vi "CANopenReadEncoder.vi"() -> ()   [LabVIEW 2020]
uses:
  <vilib>/Platform/TimedLoop/XDataNode/timing_clust.ctl
  <vilib>/Platform/TimedLoop/XDataNode/nitl_modes.ctl
  <vilib>/Platform/TimedLoop/XDataNode/wakeup.ctl
  <vilib>/CANopenLib/CANOPEN.llb/CANopen Interface Create.vi
  <vilib>/CANopenLib/CANOPEN.llb/CANopen TPDO Create.vi
  <vilib>/CANopenLib/CANOPEN.llb/CANopen TPDO Start.vi
  <vilib>/CANopenLib/CANOPEN.llb/CANopen SDO Create.vi
  <vilib>/CANopenLib/CANOPEN.llb/CANopen SDO Write [I16].vi
  <vilib>/CANopenLib/CANOPEN.llb/CANopen SDO Close.vi
  <vilib>/CANopenLib/CANOPEN.llb/CANopen SYNC Create.vi
  <vilib>/CANopenLib/CANOPEN.llb/CANopen RPDO Create.vi
  <vilib>/CANopenLib/CANOPEN.llb/CANopen SYNC Start.vi
  <vilib>/CANopenLib/CANOPEN.llb/CANopen RPDO Start.vi
  <vilib>/CANopenLib/CANOPEN.llb/CANopen Fetch from Data [U32].vi
  <vilib>/CANopenLib/CANOPEN.llb/CANopen TPDO Close.vi
  <vilib>/CANopenLib/CANOPEN.llb/CANopen Interface Close.vi
  <vilib>/CANopenLib/CANOPEN.llb/CANopen Convert To Data [I16].vi
  <vilib>/CANopenLib/CANOPEN.llb/CANopen Fetch from Data [I16].vi
  <vilib>/CANopenLib/CANOPEN.llb/CANopen Fetch from Data [I32].vi
  <vilib>/CANopenLib/CANOPEN.llb/CANopen SYNC Close.vi
  <vilib>/CANopenLib/CANOPEN.llb/CANopen RPDO Close.vi
  <vilib>/Platform/TimedLoop/XDataNode/XDataNode.xnode
  <vilib>/Platform/TimedLoop/XDataNode/XDNodeRunTimeDep.lvlib
panel:
  out "Target_Speed2":dbl
  out "Target_Speed1":dbl
  out "completion code 5":u32
  in  "buffer size (0) 7":u16
  in  "TPDO channel 2":u8(ring)=2 items=["PDO 1", "PDO 2", "PDO 3", "PDO 4"]
  in  "Set Target Vilocity 2":i16
  in  "stop 5":bool
  out "timestamp 5":timestamp=timestamp(3829477264.1142135 s since 1904-01-01)
  out "电机绝对位置 2":i32=2114697600
  out "速度反馈值 2":i32
  out "转矩反馈值 0.1% 2":i16=-28
  in  "buffer size (0) 6":u16=10
  in  "TPDO channel read 2":u8(ring)=1 items=["PDO 1", "PDO 2", "PDO 3", "PDO 4"]
  in  "RPDO channel write 2":u8(ring)=1 items=["PDO 1", "PDO 2", "PDO 3", "PDO 4"]
  in  "period (ms) 5":i64=10
  out "completion code 4":u32
  out "completion code 3":u32
  in  "batch SDO name 2":string="Nimotion_VM"
  in  "node-ID  2":u8=2 min=1 max=127 step=1
  out "completion code":u32
  in  "buffer size (0) 5":u16
  in  "TPDO channel":u8(ring)=2 items=["PDO 1", "PDO 2", "PDO 3", "PDO 4"]
  in  "Set Target Vilocity":i16
  in  "stop 4":bool
  out "timestamp 4":timestamp=timestamp(3829477264.1140933 s since 1904-01-01)
  out "电机绝对位置":i32=-1267158272
  out "速度反馈值":i32
  out "转矩反馈值 0.1%":i16=-12
  in  "buffer size (0) 4":u16=10
  in  "TPDO channel read":u8(ring)=1 items=["PDO 1", "PDO 2", "PDO 3", "PDO 4"]
  in  "RPDO channel write":u8(ring)=1 items=["PDO 1", "PDO 2", "PDO 3", "PDO 4"]
  in  "period (ms) 4":i64=10
  out "completion code 2":u32
  out "completion code 1":u32
  in  "batch SDO name":string="Nimotion_VM"
  in  "node-ID  4":u8=1 min=1 max=127 step=1
  in  "baud rate 2":u32(ring) items=["1 Mbit/s"=0, "800 kbit/s"=1, "500 kbit/s"=2, "250 kbit/s"=3, "125 kbit/s"=4, "50 kbit/s"=6, "20 kbit/s"=7, "10 kbit/s"=8]
  in  "CANopen interface 2":u32(ring) items=["CANopen01", "CANopen02", "CANopen03", "CANopen04", "CANopen05", "CANopen06", "CANopen07", "CANopen08", "CANopen09", "CANopen10", "CANopen11", "CANopen12", "CANopen13", "CANopen14", "CANopen15", "CANopen16", "CANopen17", "CANopen18", "CANopen19", "CANopen20", "CANopen21", "CANopen22", "CANopen23", "CANopen24", "CANopen25", "CANopen26", "CANopen27", "CANopen28", "CANopen29", "CANopen30", "CANopen31", "CANopen32"]
  in  "buffer size (0) 3":u16=10
  in  "period (ms) 3":i64=1
  in  "stop 3":bool
  out "New data? 3":bool
  out "timestamp 3":timestamp
  out "当前位置 3":u32
  out "基座原始角度值":dbl
  out "TPDO Data 3":u8[](array[numeric])
  out "基座角度值":dbl
  in  "PDO channel 3":u8(ring) items=["PDO 1", "PDO 2", "PDO 3", "PDO 4"]
  in  "node-ID 3":u8=3 min=1 max=127 step=1
  in  "buffer size (0) 2":u16=10
  in  "period (ms) 2":i64=1
  in  "stop 2":bool
  out "New data? 2":bool
  out "timestamp 2":timestamp
  out "当前位置 2":u32
  out "大臂原始角度值":dbl
  out "TPDO Data 2":u8[](array[numeric])
  out "大臂角度值":dbl
  in  "PDO channel 2":u8(ring) items=["PDO 1", "PDO 2", "PDO 3", "PDO 4"]
  in  "node-ID 2":u8=2 min=1 max=127 step=1
  out "三角形角度":dbl
  out "手腕角度值":dbl
  out "TPDO Data":u8[](array[numeric])
  out "手腕原始角度值":dbl
  out "当前位置":u32
  in  "buffer size (0)":u16=10
  in  "period (ms)":i64=1
  in  "stop":bool
  out "New data?":bool
  out "timestamp":timestamp
  in  "PDO channel":u8(ring) items=["PDO 1", "PDO 2", "PDO 3", "PDO 4"]
  in  "node-ID":u8=1 min=1 max=127 step=1
  in  "baud rate":u32(ring)=2 items=["1 Mbit/s"=0, "800 kbit/s"=1, "500 kbit/s"=2, "250 kbit/s"=3, "125 kbit/s"=4, "50 kbit/s"=6, "20 kbit/s"=7, "10 kbit/s"=8]
  in  "CANopen interface":u32(ring)=2 items=["CANopen01", "CANopen02", "CANopen03", "CANopen04", "CANopen05", "CANopen06", "CANopen07", "CANopen08", "CANopen09", "CANopen10", "CANopen11", "CANopen12", "CANopen13", "CANopen14", "CANopen15", "CANopen16", "CANopen17", "CANopen18", "CANopen19", "CANopen20", "CANopen21", "CANopen22", "CANopen23", "CANopen24", "CANopen25", "CANopen26", "CANopen27", "CANopen28", "CANopen29", "CANopen30", "CANopen31", "CANopen32"]
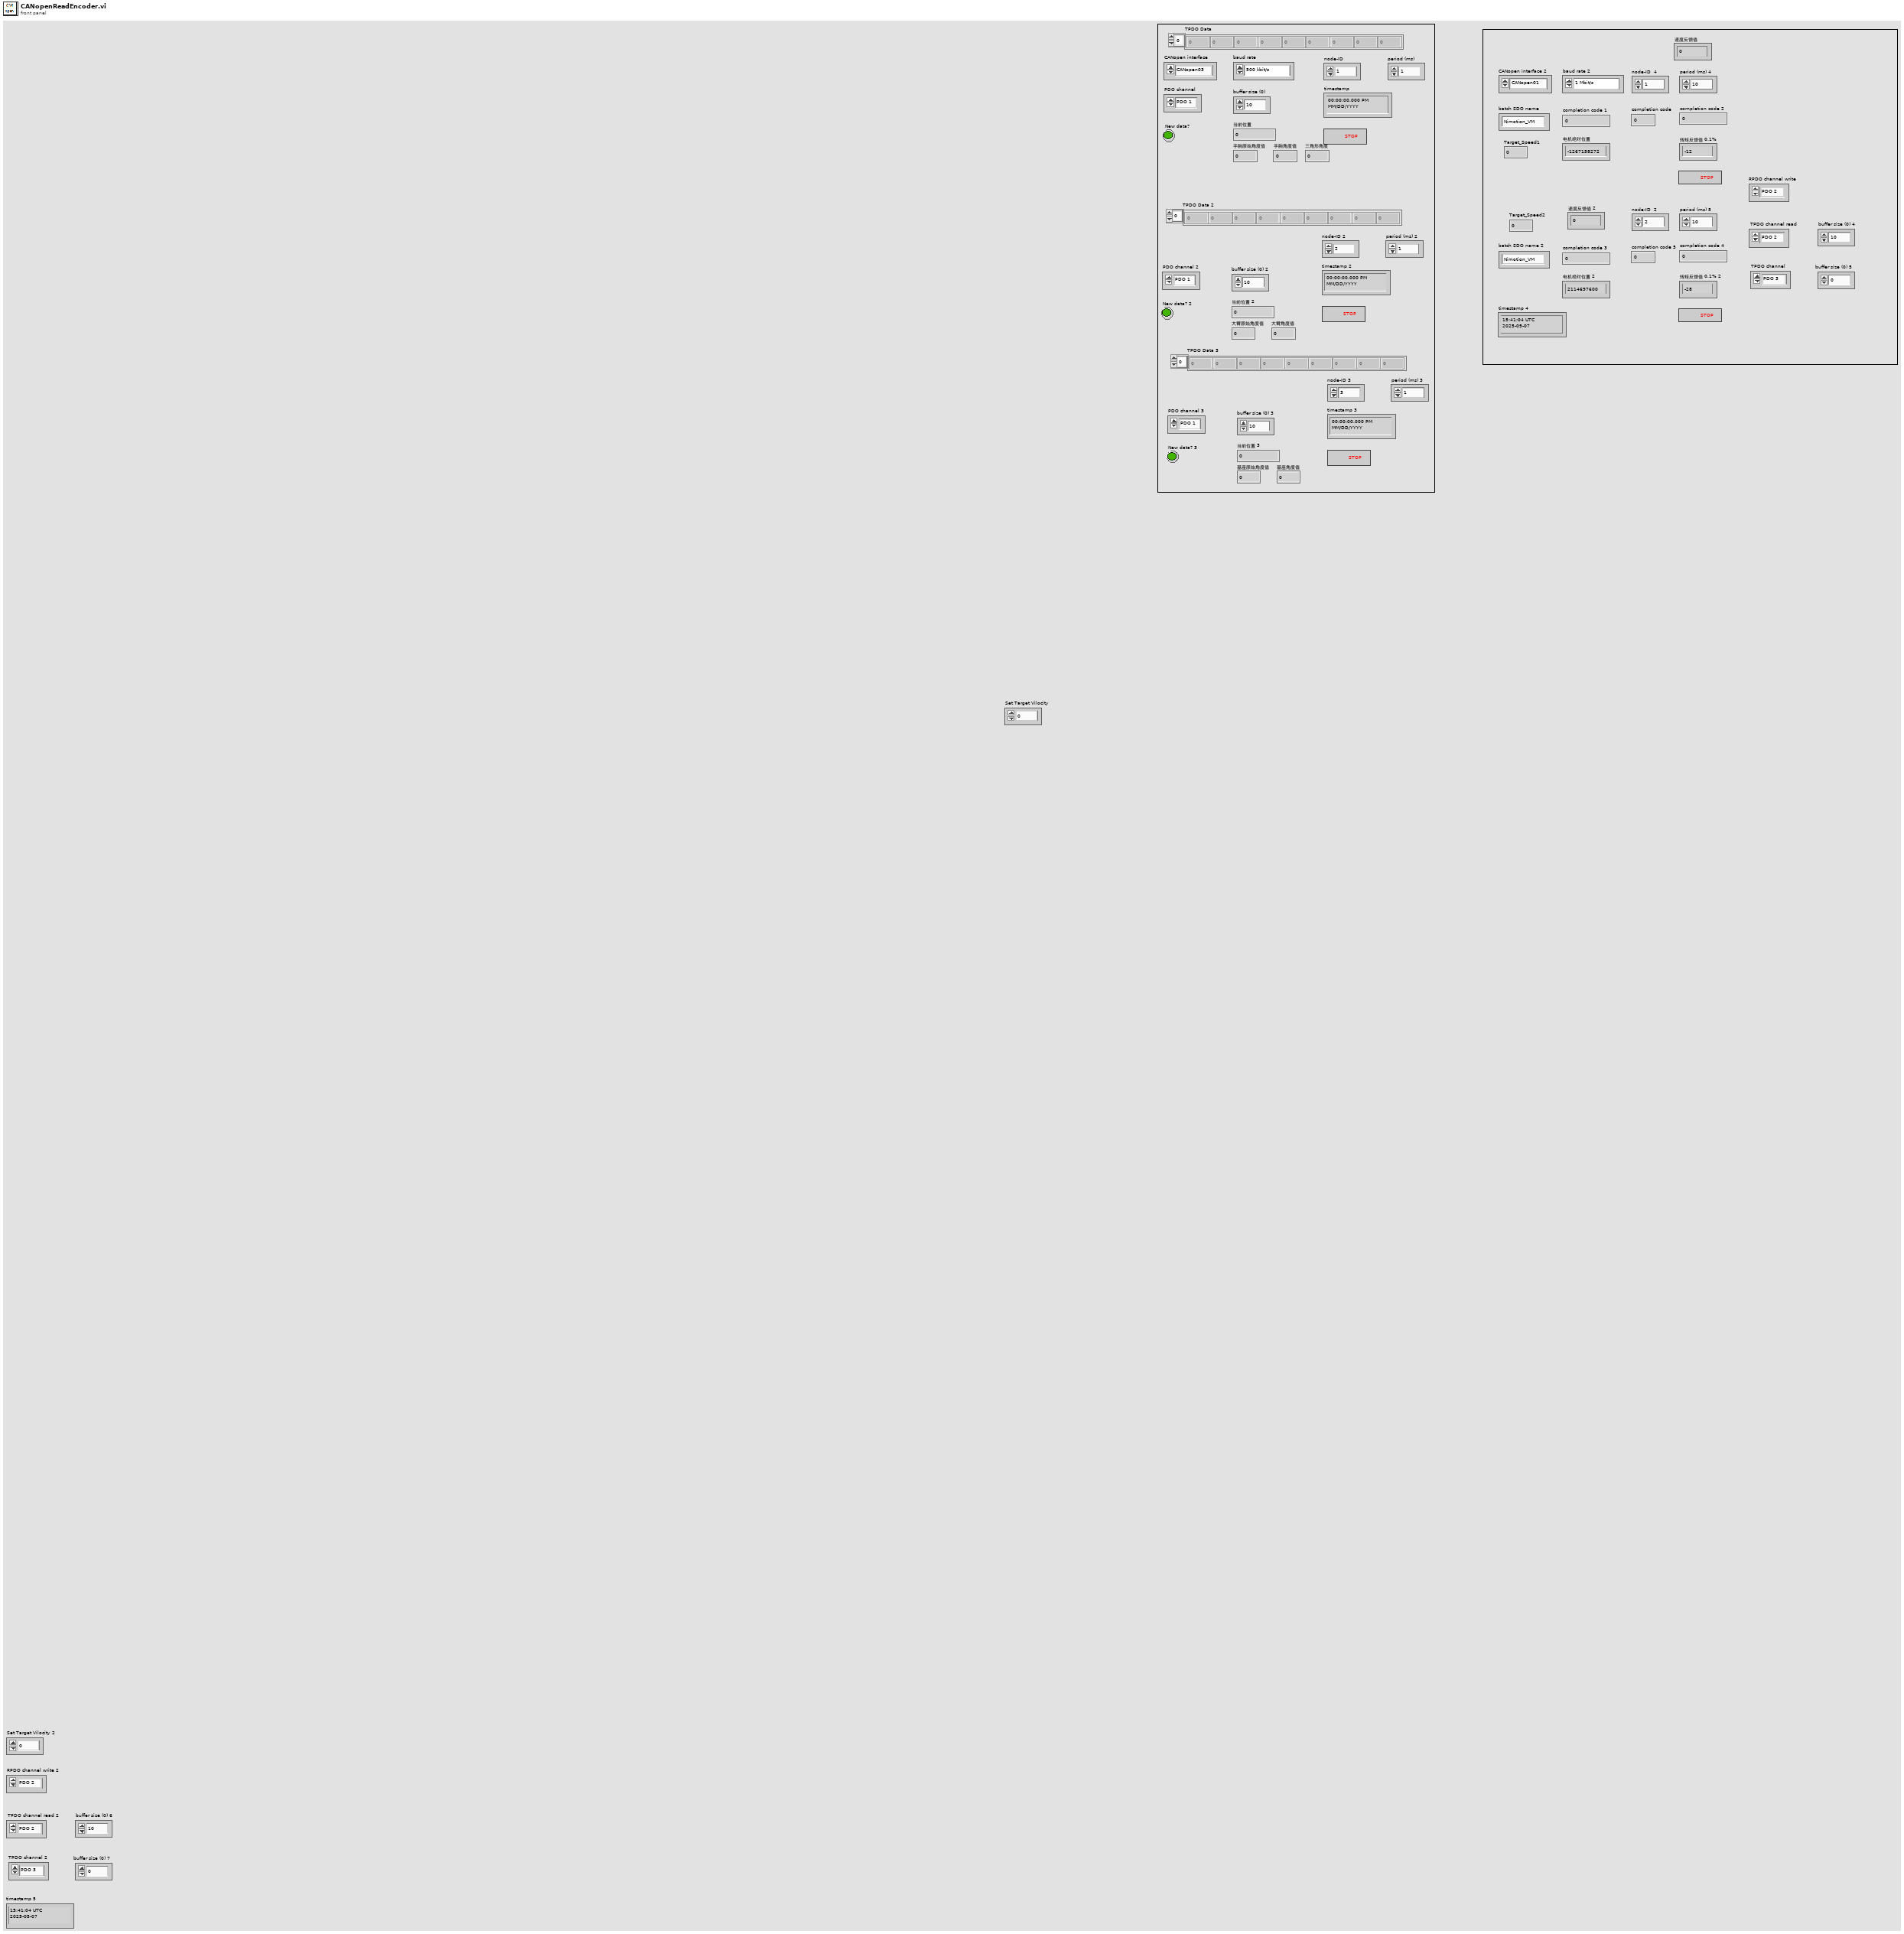
[diagram p1: front panel]
types:
  T1 = typedef "XDNodeRunTimeDep.lvlib/timing_clust.ctl" = cluster{"Expected End [f-1]":u64, "Actual End [f-1]":u64, "Finished Late? [f-1]":bool, "Expected End [i-1]":u64, "Actual End [i-1]":u64, "Finished Late? [i-1]":bool, "Expected Start [i]":u64, "Actual Start [i]":u64, "Expected Start [f]":u64, "Actual Start [f]":u64, "Source Name":string, "Structure Name":string, "Period":i64, "Deadline":i64, "Offset":i64, "Start":i64, "Priority":i32, "Timeout":i32, "Mode":T2, "Wakeup Reason":T3, "Error":errorcluster, "Source Type":string, "Secondary Source Type":string, "Global End Time":u64, "Global Start Time":u64, "Frame Duration":u64, "Iteration Duration":u64, "Assigned CPU":i32, "I/O Scan Engine Mode":u32}
  T2 = typedef "XDNodeRunTimeDep.lvlib/nitl_modes.ctl" = enum32{"No Change", "Process missed periods, maintain original phase", "Discard missed periods, maintain original phase", "Process missed periods, ignore original phase", "Discard missed periods, ignore original phase"}
  T3 = typedef "XDNodeRunTimeDep.lvlib/wakeup.ctl" = enum32{"Normal", "Aborted", "Asynchronous wakeup", "Timing source error", "Timed loop error", "Timeout"}
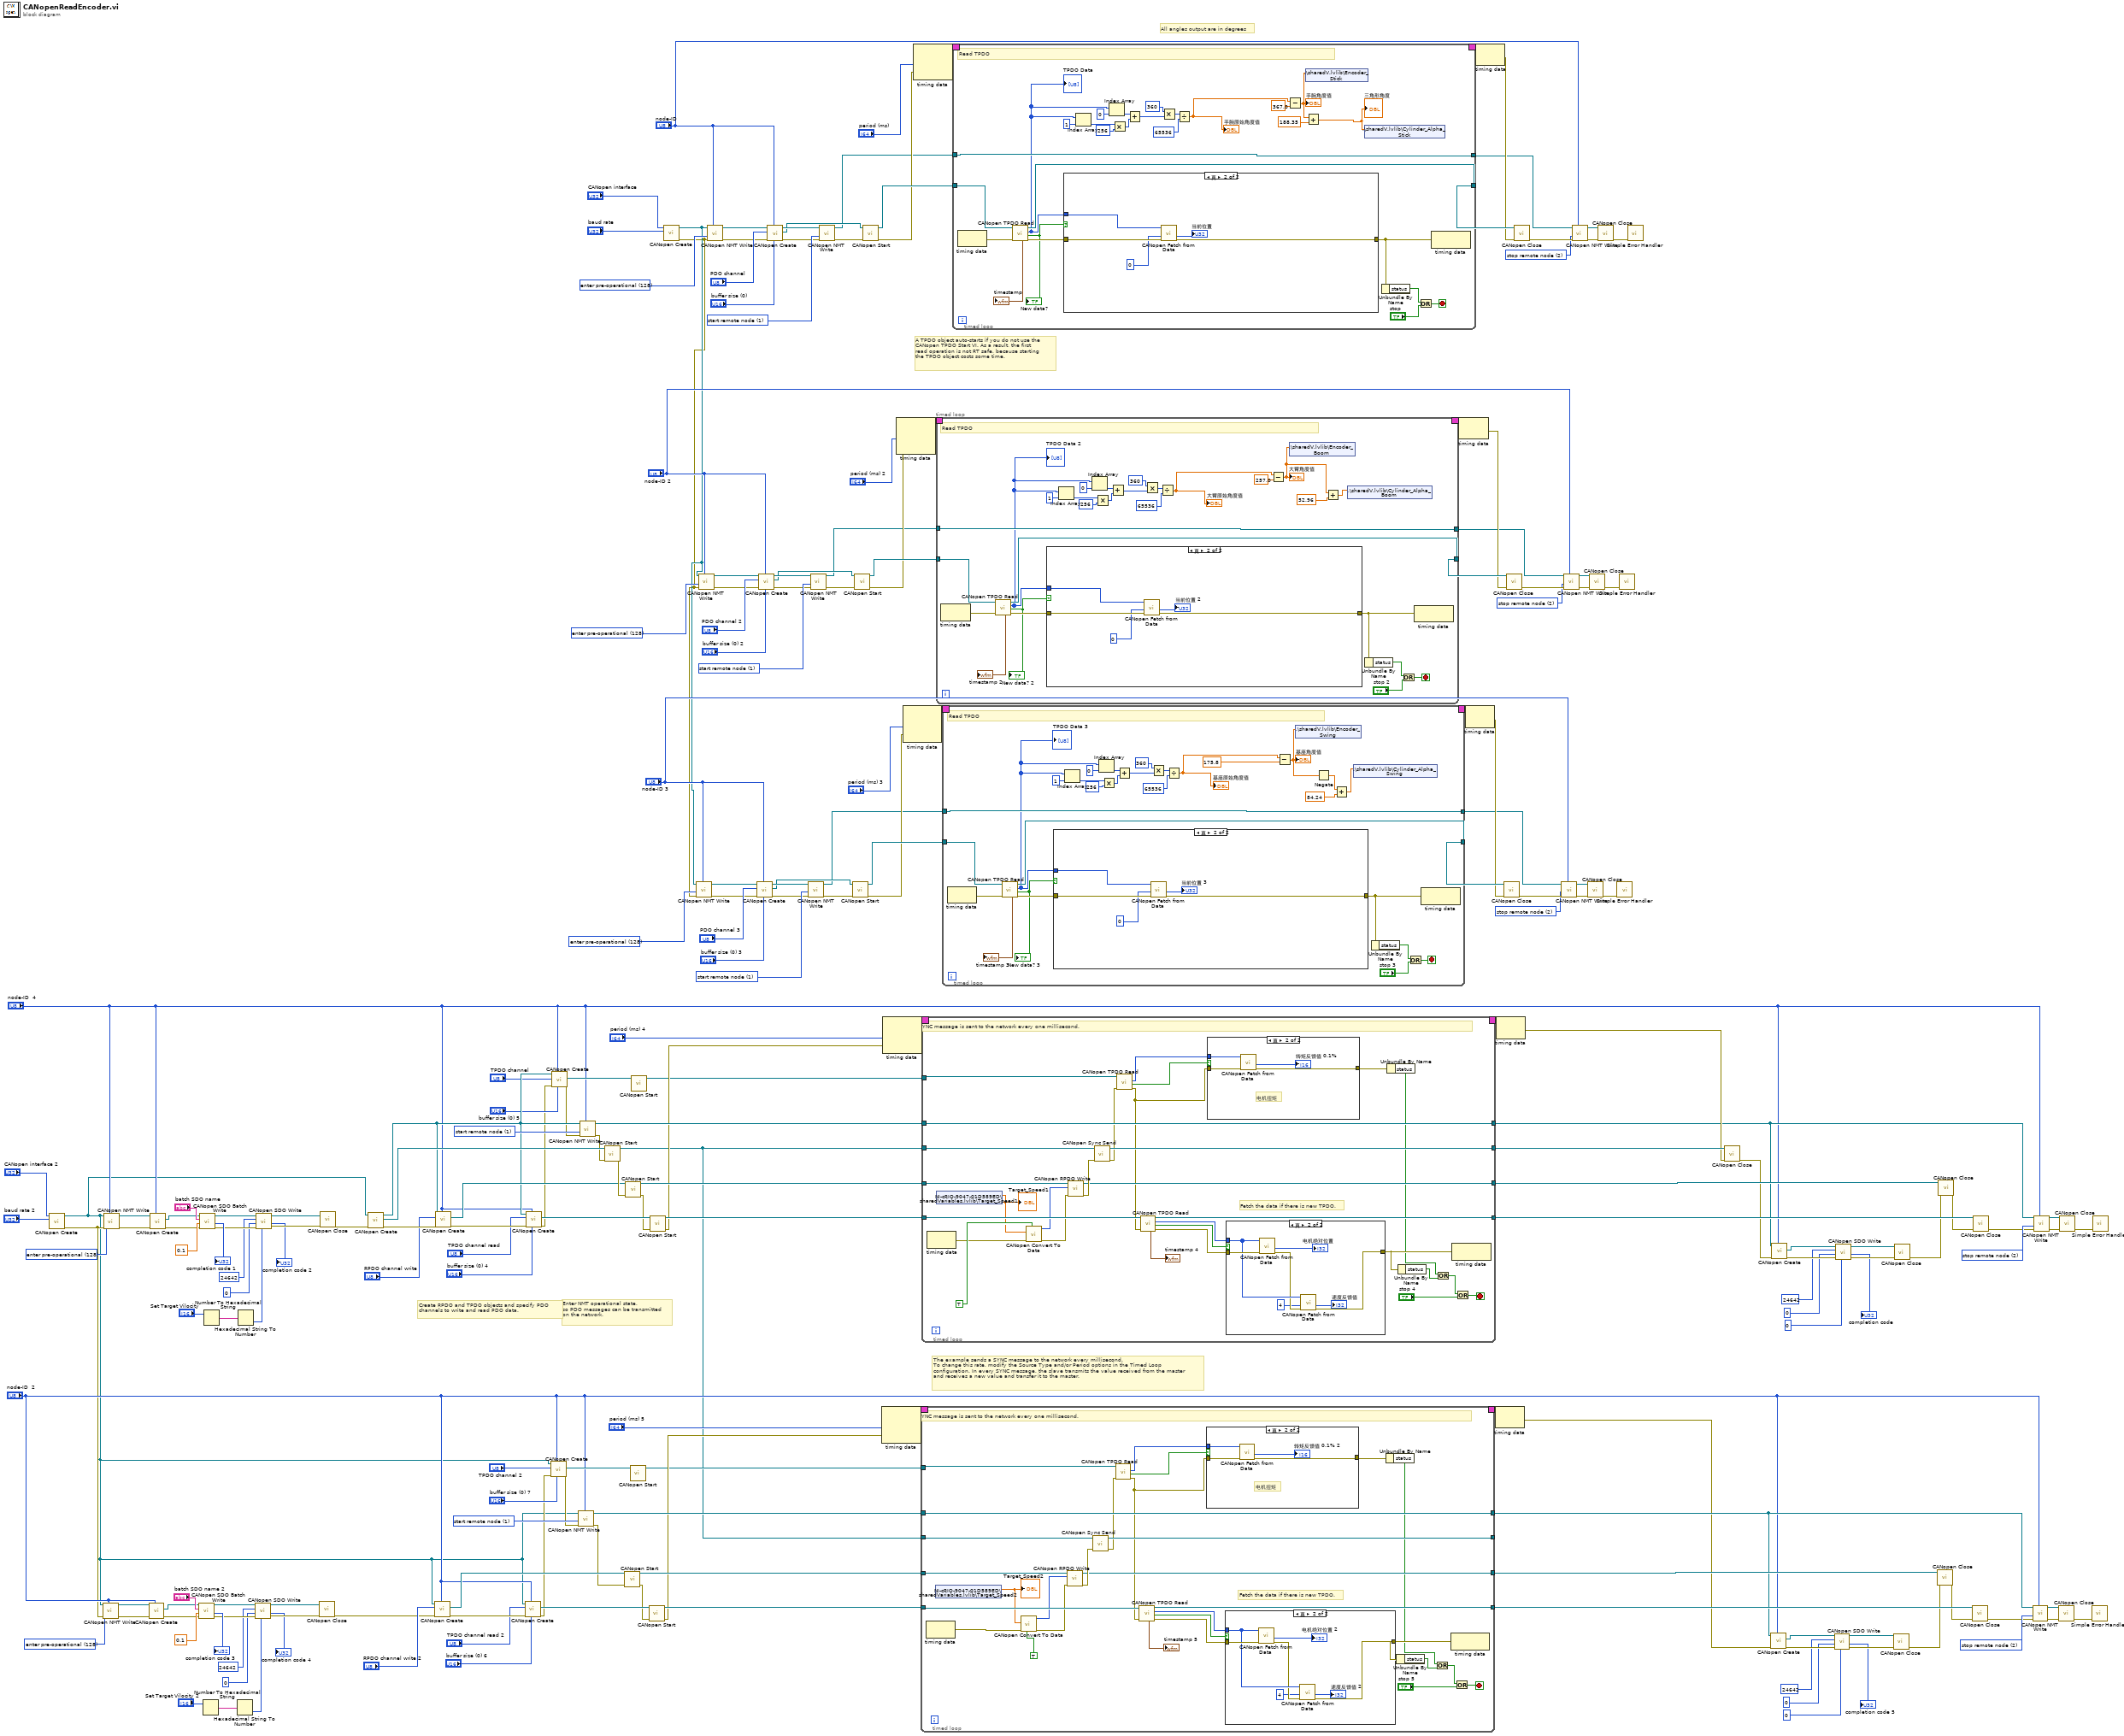
[diagram p0: block diagram]
diagram:
  w38 = u16 2 items=["start remote node"=1, "stop remote node"=2, "enter pre-operational"=128, "reset node"=129, "reset communication"=130] ("command")
  w46 = u16 1 items=["start remote node"=1, "stop remote node"=2, "enter pre-operational"=128, "reset node"=129, "reset communication"=130] ("command")
  w60 = u16 128 items=["start remote node"=1, "stop remote node"=2, "enter pre-operational"=128, "reset node"=129, "reset communication"=130] ("command")
  w98 = u16 2 items=["start remote node"=1, "stop remote node"=2, "enter pre-operational"=128, "reset node"=129, "reset communication"=130] ("command")
  w109 = u16 1 items=["start remote node"=1, "stop remote node"=2, "enter pre-operational"=128, "reset node"=129, "reset communication"=130] ("command")
  w125 = u16 128 items=["start remote node"=1, "stop remote node"=2, "enter pre-operational"=128, "reset node"=129, "reset communication"=130] ("command")
  w148 = u16 1 items=["start remote node"=1, "stop remote node"=2, "enter pre-operational"=128, "reset node"=129, "reset communication"=130] ("command")
  w152 = u16 2 items=["start remote node"=1, "stop remote node"=2, "enter pre-operational"=128, "reset node"=129, "reset communication"=130] ("command")
  w159 = u16 128 items=["start remote node"=1, "stop remote node"=2, "enter pre-operational"=128, "reset node"=129, "reset communication"=130] ("command")
  w173 = u16 1 items=["start remote node"=1, "stop remote node"=2, "enter pre-operational"=128, "reset node"=129, "reset communication"=130] ("command")
  w177 = u16 2 items=["start remote node"=1, "stop remote node"=2, "enter pre-operational"=128, "reset node"=129, "reset communication"=130] ("command")
  w184 = u16 128 items=["start remote node"=1, "stop remote node"=2, "enter pre-operational"=128, "reset node"=129, "reset communication"=130] ("command")
  w198 = u16 1 items=["start remote node"=1, "stop remote node"=2, "enter pre-operational"=128, "reset node"=129, "reset communication"=130] ("command")
  w202 = u16 2 items=["start remote node"=1, "stop remote node"=2, "enter pre-operational"=128, "reset node"=129, "reset communication"=130] ("command")
  w209 = u16 128 items=["start remote node"=1, "stop remote node"=2, "enter pre-operational"=128, "reset node"=129, "reset communication"=130] ("command")
  # "SYNC message is sent to the network every one millisecond."
  # "SYNC message is sent to the network every one millisecond."
  # "The example sends a SYNC message to the network every millisecond.\nTo change this rate, modify the Source Type and/or Period options in the Timed Loop\nconfiguration. In every SYNC message, the slave transmits the value received from the master\nand receives a new value and transfer it to the master."
  # "Enter NMT operational state,\nso PDO messages can be transmitted\non the network."
  # "Create RPDO and TPDO objects and specify PDO \nchannels to write and read PDO data."
  # "All angles output are in degrees"
  # "A TPDO object auto-starts if you do not use the \nCANopen TPDO Start VI. As a result, the first \nread operation is not RT safe, because starting \nthe TPDO object costs some time."
  n1 = call-poly <vilib>:"CANopen Create.vi"("baud rate"="baud rate 2", "interface name"="CANopen interface 2") -> ("error out"=w6:errorcluster, "interface object out"=w2:refnum<k20>)  [unwired: 8 in]
  n2 = call <vilib>:"CANopen NMT Write.vi"("node-ID (0)"="node-ID  2", "error in (no error)"=w6, "command"=w60, "interface object in"=w2) -> ("error out"=w61:errorcluster, "interface object out"=w62:refnum<k20>)  [unwired: 6 in]
  n3 = call <vilib>:"CANopen NMT Write.vi"("node-ID (0)"="node-ID  4", "error in (no error)"=w6, "command"=w125, "interface object in"=w2) -> ("error out"=w128:errorcluster, "interface object out"=w129:refnum<k20>)  [unwired: 6 in]
  n4 = call-poly <vilib>:"CANopen Create.vi"("node-ID"="node-ID  2", "error in (no error)"=w61, "interface object in"=w62) -> ("error out"=w51:errorcluster, "SDO object out"=w57:refnum<k20>)  [unwired: 6 in, 1 out]
  n5 = call-poly <vilib>:"CANopen Create.vi"("node-ID"="node-ID  4", "error in (no error)"=w128, "interface object in"=w129) -> ("error out"=w116:errorcluster, "SDO object out"=w122:refnum<k20>)  [unwired: 6 in, 1 out]
  n6 = call <vilib>:"CANopen SDO Batch Write.vi"("error in (no error)"=w51, "timeout (1s)"=0.1 ("timeout (0s)"), "batch SDO name"="batch SDO name 2", "SDO object in"=w57) -> ("error out"=w52:errorcluster, "completion code"=→"completion code 3":u32, "SDO object out"=w55:refnum<k20>)  [unwired: 5 in]
  n7 = call <vilib>:"CANopen SDO Batch Write.vi"("error in (no error)"=w116, "timeout (1s)"=0.1 ("timeout (0s)"), "batch SDO name"="batch SDO name", "SDO object in"=w122) -> ("error out"=w117:errorcluster, "completion code"=→"completion code 1":u32, "SDO object out"=w120:refnum<k20>)  [unwired: 5 in]
  n8 = Number To Hexadecimal String(2:"Set Target Vilocity 2") -> (0:w28:string)  [unwired: 1 in]
  n9 = Number To Hexadecimal String(2:"Set Target Vilocity") -> (0:w86:string)  [unwired: 1 in]
  n10 = Hexadecimal String To Number(string=w28) -> (number=w26:u32)  [unwired: 2 in, 1 out]
  n11 = Hexadecimal String To Number(string=w86) -> (number=w84:u32)  [unwired: 2 in, 1 out]
  n12 = call-poly <vilib>:"CANopen SDO Write.vi"("I16 data"=w26, "error in (no error)"=w52, "object sub-index (0)"=u8 0, "object index"=u16 24642, "SDO object in"=w55) -> ("error out"=w53:errorcluster, "completion code"=→"completion code 4":u32, "SDO object out"=w54:refnum<k20>)  [unwired: 4 in]
  n13 = call-poly <vilib>:"CANopen SDO Write.vi"("I16 data"=w84, "error in (no error)"=w117, "object sub-index (0)"=u8 0, "object index"=u16 24642, "SDO object in"=w120) -> ("error out"=w118:errorcluster, "completion code"=→"completion code 2":u32, "SDO object out"=w119:refnum<k20>)  [unwired: 4 in]
  n14 = call-poly <vilib>:"CANopen Close.vi"("error in (no error)"=w53, "SDO object in"=w54) -> ("error out"=w5:errorcluster)  [unwired: 9 in]
  n15 = call-poly <vilib>:"CANopen Close.vi"("error in (no error)"=w118, "SDO object in"=w119) -> ("error out"=w101:errorcluster)  [unwired: 9 in]
  n16 = call-poly <vilib>:"CANopen Create.vi"("error in (no error)"=w101, "interface object in"=w2) -> ("error out"=w111:errorcluster, "SYNC object out"=w110:refnum<k20>, "interface object out"=w82:refnum<k20>)  [unwired: 7 in]
  n17 = call-poly <vilib>:"CANopen Create.vi"("node-ID"="node-ID  2", "error in (no error)"=w5, "PDO channel"="RPDO channel write 2", "interface object in"=w2) -> ("error out"=w44:errorcluster, "RPDO object out"=w43:refnum<k20>)  [unwired: 5 in, 1 out]
  n18 = call-poly <vilib>:"CANopen Create.vi"("node-ID"="node-ID  4", "error in (no error)"=w111, "PDO channel"="RPDO channel write", "interface object in"=w82) -> ("error out"=w105:errorcluster, "RPDO object out"=w104:refnum<k20>)  [unwired: 5 in, 1 out]
  n19 = call-poly <vilib>:"CANopen Create.vi"("buffer size (0)"="buffer size (0) 6", "node-ID"="node-ID  2", "error in (no error)"=w44, "PDO channel"="TPDO channel read 2", "interface object in"=w2) -> ("error out"=w20:errorcluster, "TPDO object out"=w48:refnum<k20>)  [unwired: 4 in, 1 out]
  n20 = call-poly <vilib>:"CANopen Create.vi"("buffer size (0)"="buffer size (0) 4", "node-ID"="node-ID  4", "error in (no error)"=w105, "PDO channel"="TPDO channel read", "interface object in"=w82) -> ("error out"=w77:errorcluster, "TPDO object out"=w113:refnum<k20>)  [unwired: 4 in, 1 out]
  n21 = call-poly <vilib>:"CANopen Create.vi"("buffer size (0)"="buffer size (0) 7", "node-ID"="node-ID  2", "error in (no error)"=w20, "PDO channel"="TPDO channel 2", "interface object in"=w2) -> ("error out"=w19:errorcluster, "TPDO object out"=w22:refnum<k20>)  [unwired: 4 in, 1 out]
  n22 = call-poly <vilib>:"CANopen Create.vi"("buffer size (0)"="buffer size (0) 5", "node-ID"="node-ID  4", "error in (no error)"=w77, "PDO channel"="TPDO channel", "interface object in"=w82) -> ("error out"=w76:errorcluster, "TPDO object out"=w79:refnum<k20>)  [unwired: 4 in, 1 out]
  n23 = call <vilib>:"CANopen NMT Write.vi"("node-ID (0)"="node-ID  2", "error in (no error)"=w19, "command"=w46, "interface object in"=w2) -> ("error out"=w4:errorcluster, "interface object out"=w32:refnum<k20>)  [unwired: 6 in]
  n24 = call <vilib>:"CANopen NMT Write.vi"("node-ID (0)"="node-ID  4", "error in (no error)"=w76, "command"=w109, "interface object in"=w82) -> ("error out"=w108:errorcluster, "interface object out"=w90:refnum<k20>)  [unwired: 6 in]
  n25 = call-poly <vilib>:"CANopen Start.vi"("error in (no error)"=w108, "SYNC object in"=w110) -> ("error out"=w107:errorcluster, "SYNC object out"=w3:refnum<k20>)  [unwired: 8 in]
  n26 = call-poly <vilib>:"CANopen Start.vi"("error in (no error)"=w4, "RPDO object in"=w43) -> ("error out"=w45:errorcluster, "RPDO object out"=w31:refnum<k20>)  [unwired: 8 in]
  n27 = call-poly <vilib>:"CANopen Start.vi"("error in (no error)"=w107, "RPDO object in"=w104) -> ("error out"=w106:errorcluster, "RPDO object out"=w89:refnum<k20>)  [unwired: 8 in]
  n28 = call-poly <vilib>:"CANopen Start.vi"("TPDO object in"=w22) -> ("TPDO object out"=w21:refnum<k20>)  [unwired: 9 in, 1 out]
  n29 = call-poly <vilib>:"CANopen Start.vi"("TPDO object in"=w79) -> ("TPDO object out"=w78:refnum<k20>)  [unwired: 9 in, 1 out]
  n30 = call-poly <vilib>:"CANopen Start.vi"("error in (no error)"=w45, "TPDO object in"=w48) -> ("error out"=w29:errorcluster, "TPDO object out"=w30:refnum<k20>)  [unwired: 8 in]
  n31 = call-poly <vilib>:"CANopen Start.vi"("error in (no error)"=w106, "TPDO object in"=w113) -> ("error out"=w87:errorcluster, "TPDO object out"=w88:refnum<k20>)  [unwired: 8 in]
  n32 = call-poly <vilib>:"CANopen Create.vi"("baud rate"="baud rate", "interface name"="CANopen interface") -> ("error out"=w134:errorcluster, "interface object out"=w135:refnum<k20>)  [unwired: 8 in]
  n33 = call <vilib>:"CANopen NMT Write.vi"("node-ID (0)"="node-ID 3", "error in (no error)"=w134, "command"=w159, "interface object in"=w135) -> ("error out"=w138:errorcluster, "interface object out"=w139:refnum<k20>)  [unwired: 6 in]
  n34 = call <vilib>:"CANopen NMT Write.vi"("node-ID (0)"="node-ID 2", "error in (no error)"=w134, "command"=w184, "interface object in"=w135) -> ("error out"=w163:errorcluster, "interface object out"=w164:refnum<k20>)  [unwired: 6 in]
  n35 = call <vilib>:"CANopen NMT Write.vi"("node-ID (0)"="node-ID", "error in (no error)"=w134, "command"=w209, "interface object in"=w135) -> ("error out"=w188:errorcluster, "interface object out"=w189:refnum<k20>)  [unwired: 6 in]
  n36 = call-poly <vilib>:"CANopen Create.vi"("buffer size (0)"="buffer size (0) 3", "node-ID"="node-ID 3", "error in (no error)"=w138, "PDO channel"="PDO channel 3", "interface object in"=w139) -> ("error out"=w146:errorcluster, "TPDO object out"=w145:refnum<k20>, "interface object out"=w149:refnum<k20>)  [unwired: 4 in]
  n37 = call-poly <vilib>:"CANopen Create.vi"("buffer size (0)"="buffer size (0) 2", "node-ID"="node-ID 2", "error in (no error)"=w163, "PDO channel"="PDO channel 2", "interface object in"=w164) -> ("error out"=w171:errorcluster, "TPDO object out"=w170:refnum<k20>, "interface object out"=w174:refnum<k20>)  [unwired: 4 in]
  n38 = call-poly <vilib>:"CANopen Create.vi"("buffer size (0)"="buffer size (0)", "node-ID"="node-ID", "error in (no error)"=w188, "PDO channel"="PDO channel", "interface object in"=w189) -> ("error out"=w196:errorcluster, "TPDO object out"=w195:refnum<k20>, "interface object out"=w199:refnum<k20>)  [unwired: 4 in]
  n39 = call <vilib>:"CANopen NMT Write.vi"("error in (no error)"=w146, "command"=w148, "interface object in"=w149) -> ("error out"=w147:errorcluster, "interface object out"=w141:refnum<k20>)  [unwired: 7 in]
  n40 = call <vilib>:"CANopen NMT Write.vi"("error in (no error)"=w171, "command"=w173, "interface object in"=w174) -> ("error out"=w172:errorcluster, "interface object out"=w166:refnum<k20>)  [unwired: 7 in]
  n41 = call <vilib>:"CANopen NMT Write.vi"("error in (no error)"=w196, "command"=w198, "interface object in"=w199) -> ("error out"=w197:errorcluster, "interface object out"=w191:refnum<k20>)  [unwired: 7 in]
  n42 = call-poly <vilib>:"CANopen Start.vi"("error in (no error)"=w147, "TPDO object in"=w145) -> ("error out"=w144:errorcluster, "TPDO object out"=w156:refnum<k20>)  [unwired: 8 in]
  n43 = call-poly <vilib>:"CANopen Start.vi"("error in (no error)"=w172, "TPDO object in"=w170) -> ("error out"=w169:errorcluster, "TPDO object out"=w181:refnum<k20>)  [unwired: 8 in]
  n44 = call-poly <vilib>:"CANopen Start.vi"("error in (no error)"=w197, "TPDO object in"=w195) -> ("error out"=w194:errorcluster, "TPDO object out"=w206:refnum<k20>)  [unwired: 8 in]
  n45 = node-c288("period (ms) 5", w29) -> (w131:T1)  [unwired: 1 in]
  n46 = node-c288("period (ms) 4", w87) -> (w133:T1)  [unwired: 1 in]
  n47 = node-c288("period (ms) 2", w169) -> (w186:T1)  [unwired: 1 in]
  n48 = node-c288("period (ms) 3", w144) -> (w161:T1)  [unwired: 1 in]
  n49 = node-c288("period (ms)", w194) -> (w212:T1)  [unwired: 1 in]
  n50 = timed-loop {
    timing: w131 -> [_]
    timing-out: [_] -> w130
    tunnel: [w231] -> _
    tunnel: [w241] -> w17
    tunnel: w32 -> [w241]
    tunnel: w31 -> [w235]
    tunnel: w30 -> [w236]
    tunnel: [w233] -> w37
    tunnel: [w232] -> w18
    tunnel: w21 -> [w224]
    tunnel: w3 -> [w214]
    stop <- w240 stop-if-true
    # "Fetch the data if there is new TPDO."
    n51 = node-c288() -> (w226:errorcluster)  [unwired: 1 in]
    n52 = shared-variable "NI-cRIO-9047-01D589ED\\sharedVariables.lvlib\\Target_Speed2"() -> (w213:dbl)  [unwired: 1 in, 1 out]
    "Target_Speed2" <- w213
    n53 = call-poly <vilib>:"CANopen Convert To Data.vi"("trim"=TRUE, "error in (no error)"=w226, "signed 16-bit integer"=w213) -> ("error out"=w215:errorcluster, "CANopen data out"=w225:u8[])  [unwired: 7 in]
    n54 = call <vilib>:"CANopen RPDO Write.vi"("error in (no error)"=w215, "data"=w225, "RPDO object in"=w235) -> ("error out"=w234:errorcluster, "RPDO object out"=w232:refnum<k20>)  [unwired: 7 in]
    n55 = call <vilib>:"CANopen Sync Send.vi"("error in (no error)"=w234, "SYNC object in"=w214) -> ("error out"=w223:errorcluster, "SYNC object out"=w231:refnum<k20>)  [unwired: 8 in]
    n56 = call <vilib>:"CANopen TPDO Read.vi"("error in (no error)"=w223, "TPDO object in"=w224) -> ("error out"=w220:errorcluster, "new data?"=w221:bool, "data"=w222:u8[])  [unwired: 5 in, 2 out]
    n57 = call <vilib>:"CANopen TPDO Read.vi"("error in (no error)"=w220, "TPDO object in"=w236) -> ("error out"=w237:errorcluster, "new data?"=w230:bool, "data"=w228:u8[], "TPDO object out"=w233:refnum<k20>, "timestamp"=→"timestamp 5":timestamp)  [unwired: 5 in]
    n58 = case shown="真" w221 {
      tunnel: w220 -> [w242 w246]
      tunnel: w222 -> [_ w245]
      tunnel: [w242 w244] -> w219
      frame False {
      }
      frame True {
        # "电机扭矩"
        n59 = call-poly <vilib>:"CANopen Fetch from Data.vi"("error in (no error)"=w246, "CANopen data in"=w245) -> ("error out"=w244:errorcluster, "signed 16-bit integer"=→"转矩反馈值 0.1% 2":i16)  [unwired: 7 in, 1 out]
      }
    }
    n60 = case shown="真" w230 {
      tunnel: w237 -> [w252 w259]
      tunnel: w228 -> [_ w257]
      tunnel: [w252 w255] -> w229
      frame False {
      }
      frame True {
        n61 = call-poly <vilib>:"CANopen Fetch from Data.vi"("error in (no error)"=w259, "CANopen data in"=w257) -> ("error out"=w256:errorcluster, "signed 32-bit integer"=→"电机绝对位置 2":i32)  [unwired: 7 in, 1 out]
        n62 = call-poly <vilib>:"CANopen Fetch from Data.vi"("error in (no error)"=w256, "offset (0)"=u32 4, "CANopen data in"=w257) -> ("error out"=w255:errorcluster, "signed 32-bit integer"=→"速度反馈值 2":i32)  [unwired: 6 in, 1 out]
      }
    }
    n63 = Unbundle By Name(w219) -> ("status"=w217:bool)
    n64 = Unbundle By Name(w229) -> ("status"=w218:bool)
    n65 = Or(x=w217, y=w218) -> (x .or. y?=w216:bool)
    n66 = node-c288(w229) -> ()  [unwired: 1 out]
    n67 = Or(x=w216, y="stop 5") -> (x .or. y?=w240:bool)
  }
  n68 = timed-loop {
    timing: w133 -> [_]
    timing-out: [_] -> w132
    tunnel: w3 -> [w288]
    tunnel: [w277] -> w94
    tunnel: [w287] -> w74
    tunnel: w90 -> [w287]
    tunnel: w89 -> [w281]
    tunnel: w88 -> [w282]
    tunnel: [w279] -> w97
    tunnel: [w278] -> w75
    tunnel: w78 -> [w270]
    stop <- w286 stop-if-true
    # "Fetch the data if there is new TPDO."
    n69 = node-c288() -> (w272:errorcluster)  [unwired: 1 in]
    n70 = shared-variable "NI-cRIO-9047-01D589ED\\sharedVariables.lvlib\\Target_Speed1"() -> (w260:dbl)  [unwired: 1 in, 1 out]
    "Target_Speed1" <- w260
    n71 = call-poly <vilib>:"CANopen Convert To Data.vi"("trim"=TRUE, "error in (no error)"=w272, "signed 16-bit integer"=w260) -> ("error out"=w261:errorcluster, "CANopen data out"=w271:u8[])  [unwired: 7 in]
    n72 = call <vilib>:"CANopen RPDO Write.vi"("error in (no error)"=w261, "data"=w271, "RPDO object in"=w281) -> ("error out"=w280:errorcluster, "RPDO object out"=w278:refnum<k20>)  [unwired: 7 in]
    n73 = call <vilib>:"CANopen Sync Send.vi"("error in (no error)"=w280, "SYNC object in"=w288) -> ("error out"=w269:errorcluster, "SYNC object out"=w277:refnum<k20>)  [unwired: 8 in]
    n74 = call <vilib>:"CANopen TPDO Read.vi"("error in (no error)"=w269, "TPDO object in"=w270) -> ("error out"=w266:errorcluster, "new data?"=w267:bool, "data"=w268:u8[])  [unwired: 5 in, 2 out]
    n75 = call <vilib>:"CANopen TPDO Read.vi"("error in (no error)"=w266, "TPDO object in"=w282) -> ("error out"=w283:errorcluster, "new data?"=w276:bool, "data"=w274:u8[], "TPDO object out"=w279:refnum<k20>, "timestamp"=→"timestamp 4":timestamp)  [unwired: 5 in]
    n76 = case shown="真" w267 {
      tunnel: w266 -> [w289 w293]
      tunnel: w268 -> [_ w292]
      tunnel: [w289 w291] -> w265
      frame False {
      }
      frame True {
        # "电机扭矩"
        n77 = call-poly <vilib>:"CANopen Fetch from Data.vi"("error in (no error)"=w293, "CANopen data in"=w292) -> ("error out"=w291:errorcluster, "signed 16-bit integer"=→"转矩反馈值 0.1%":i16)  [unwired: 7 in, 1 out]
      }
    }
    n78 = case shown="真" w276 {
      tunnel: w283 -> [w299 w306]
      tunnel: w274 -> [_ w304]
      tunnel: [w299 w302] -> w275
      frame False {
      }
      frame True {
        n79 = call-poly <vilib>:"CANopen Fetch from Data.vi"("error in (no error)"=w306, "CANopen data in"=w304) -> ("error out"=w303:errorcluster, "signed 32-bit integer"=→"电机绝对位置":i32)  [unwired: 7 in, 1 out]
        n80 = call-poly <vilib>:"CANopen Fetch from Data.vi"("error in (no error)"=w303, "offset (0)"=u32 4, "CANopen data in"=w304) -> ("error out"=w302:errorcluster, "signed 32-bit integer"=→"速度反馈值":i32)  [unwired: 6 in, 1 out]
      }
    }
    n81 = Unbundle By Name(w265) -> ("status"=w263:bool)
    n82 = Unbundle By Name(w275) -> ("status"=w264:bool)
    n83 = Or(x=w263, y=w264) -> (x .or. y?=w262:bool)
    n84 = node-c288(w275) -> ()  [unwired: 1 out]
    n85 = Or(x=w262, y="stop 4") -> (x .or. y?=w286:bool)
  }
  n86 = timed-loop {
    tunnel: [w330] -> w183
    tunnel: w181 -> [w333]
    timing: w186 -> [_]
    timing-out: [_] -> w185
    tunnel: w166 -> [w324]
    tunnel: [w324] -> w165
    stop <- w328 stop-if-true
    # "Read TPDO"
    n87 = node-c288() -> (w326:errorcluster)  [unwired: 1 in]
    n88 = call <vilib>:"CANopen TPDO Read.vi"("error in (no error)"=w326, "TPDO object in"=w333) -> ("error out"=w331:errorcluster, "new data?"=w327:bool, "data"=w318:u8[], "TPDO object out"=w330:refnum<k20>, "timestamp"=→"timestamp 2":timestamp)  [unwired: 5 in]
    "New data? 2" <- w327
    "TPDO Data 2" <- w318
    n89 = case shown="真" w327 {
      tunnel: w331 -> [w339 w344]
      tunnel: w318 -> [_ w343]
      tunnel: [w339 w342] -> w323
      frame False {
      }
      frame True {
        n90 = call-poly <vilib>:"CANopen Fetch from Data.vi"("error in (no error)"=w344, "offset (0)"=u32 0, "CANopen data in"=w343) -> ("error out"=w342:errorcluster, "unsigned 32-bit integer"=→"当前位置 2":u32)  [unwired: 6 in, 1 out]
      }
    }
    n91 = Index Array(array=w318, index=1) -> (element=w315:u8)
    n92 = Index Array(array=w318, index=0) -> (element=w314:u8)
    n93 = Multiply(x=w315, y=256) -> (x*y=w313:i32)
    n94 = Add(x=w314, y=w313) -> (x+y=w312:i32)
    n95 = Multiply(x=u32 360, y=w312) -> (x*y=w321:u32)
    n96 = Divide(x=w321, y=u32 65536) -> (x/y=w310:dbl)
    "大臂原始角度值" <- w310
    n97 = Subtract(x=w310, y=257.0) -> (x-y=w308:dbl)
    "大臂角度值" <- w308
    n98 = shared-variable ".\\sharedV.lvlib\\Encoder_Boom"(w308) -> ()  [unwired: 1 in, 1 out]
    n99 = Add(x=w308, y=52.96) -> (x+y=w307:dbl)
    n100 = shared-variable ".\\sharedV.lvlib\\Cylinder_Alpha_Boom"(w307) -> ()  [unwired: 1 in, 1 out]
    n101 = Unbundle By Name(w323) -> ("status"=w325:bool)
    n102 = Or(x=w325, y="stop 2") -> (x .or. y?=w328:bool)
    n103 = node-c288(w323) -> ()  [unwired: 1 out]
  }
  n104 = timed-loop {
    tunnel: [w369] -> w158
    tunnel: w156 -> [w372]
    timing: w161 -> [_]
    timing-out: [_] -> w160
    tunnel: w141 -> [w363]
    tunnel: [w363] -> w140
    stop <- w367 stop-if-true
    # "Read TPDO"
    n105 = node-c288() -> (w365:errorcluster)  [unwired: 1 in]
    n106 = call <vilib>:"CANopen TPDO Read.vi"("error in (no error)"=w365, "TPDO object in"=w372) -> ("error out"=w370:errorcluster, "new data?"=w366:bool, "data"=w357:u8[], "TPDO object out"=w369:refnum<k20>, "timestamp"=→"timestamp 3":timestamp)  [unwired: 5 in]
    "New data? 3" <- w366
    "TPDO Data 3" <- w357
    n107 = case shown="真" w366 {
      tunnel: w370 -> [w378 w383]
      tunnel: w357 -> [_ w382]
      tunnel: [w378 w381] -> w362
      frame False {
      }
      frame True {
        n108 = call-poly <vilib>:"CANopen Fetch from Data.vi"("error in (no error)"=w383, "offset (0)"=u32 0, "CANopen data in"=w382) -> ("error out"=w381:errorcluster, "unsigned 32-bit integer"=→"当前位置 3":u32)  [unwired: 6 in, 1 out]
      }
    }
    n109 = Index Array(array=w357, index=1) -> (element=w354:u8)
    n110 = Index Array(array=w357, index=0) -> (element=w353:u8)
    n111 = Multiply(x=w354, y=256) -> (x*y=w352:i32)
    n112 = Add(x=w353, y=w352) -> (x+y=w351:i32)
    n113 = Multiply(x=u32 360, y=w351) -> (x*y=w360:u32)
    n114 = Divide(x=w360, y=u32 65536) -> (x/y=w349:dbl)
    "基座原始角度值" <- w349
    n115 = Subtract(x=w349, y=175.8) -> (x-y=w346:dbl)
    "基座角度值" <- w346
    n116 = shared-variable ".\\sharedV.lvlib\\Encoder_Swing"(w346) -> ()  [unwired: 1 in, 1 out]
    n117 = Negate(x=w346) -> (-x=w345:dbl)
    n118 = Add(x=w345, y=84.24) -> (x+y=w347:dbl)
    n119 = shared-variable ".\\sharedV.lvlib\\Cylinder_Alpha_Swing"(w347) -> ()  [unwired: 1 in, 1 out]
    n120 = Unbundle By Name(w362) -> ("status"=w364:bool)
    n121 = Or(x=w364, y="stop 3") -> (x .or. y?=w367:bool)
    n122 = node-c288(w362) -> ()  [unwired: 1 out]
  }
  n123 = timed-loop {
    tunnel: [w407] -> w208
    tunnel: w206 -> [w410]
    timing: w212 -> [_]
    timing-out: [_] -> w211
    tunnel: w191 -> [w401]
    tunnel: [w401] -> w190
    stop <- w405 stop-if-true
    # "Read TPDO"
    n124 = node-c288() -> (w403:errorcluster)  [unwired: 1 in]
    n125 = call <vilib>:"CANopen TPDO Read.vi"("error in (no error)"=w403, "TPDO object in"=w410) -> ("error out"=w408:errorcluster, "new data?"=w404:bool, "data"=w395:u8[], "TPDO object out"=w407:refnum<k20>, "timestamp"=→"timestamp":timestamp)  [unwired: 5 in]
    "New data?" <- w404
    "TPDO Data" <- w395
    n126 = case shown="真" w404 {
      tunnel: w408 -> [w416 w421]
      tunnel: w395 -> [_ w420]
      tunnel: [w416 w419] -> w400
      frame False {
      }
      frame True {
        n127 = call-poly <vilib>:"CANopen Fetch from Data.vi"("error in (no error)"=w421, "offset (0)"=u32 0, "CANopen data in"=w420) -> ("error out"=w419:errorcluster, "unsigned 32-bit integer"=→"当前位置":u32)  [unwired: 6 in, 1 out]
      }
    }
    n128 = Index Array(array=w395, index=1) -> (element=w392:u8)
    n129 = Index Array(array=w395, index=0) -> (element=w391:u8)
    n130 = Multiply(x=w392, y=256) -> (x*y=w390:i32)
    n131 = Add(x=w391, y=w390) -> (x+y=w389:i32)
    n132 = Multiply(x=u32 360, y=w389) -> (x*y=w398:u32)
    n133 = Divide(x=w398, y=u32 65536) -> (x/y=w387:dbl)
    "手腕原始角度值" <- w387
    n134 = Subtract(x=w387, y=367.0) -> (x-y=w385:dbl)
    "手腕角度值" <- w385
    n135 = shared-variable ".\\sharedV.lvlib\\Encoder_Stick"(w385) -> ()  [unwired: 1 in, 1 out]
    n136 = Add(x=w385, y=188.35) -> (x+y=w384:dbl)
    "三角形角度" <- w384
    n137 = shared-variable ".\\sharedV.lvlib\\Cylinder_Alpha_Stick"(w384) -> ()  [unwired: 1 in, 1 out]
    n138 = Unbundle By Name(w400) -> ("status"=w402:bool)
    n139 = Or(x=w402, y="stop") -> (x .or. y?=w405:bool)
    n140 = node-c288(w400) -> ()  [unwired: 1 out]
  }
  n141 = node-c288(w185) -> (w168:errorcluster)
  n142 = node-c288(w160) -> (w143:errorcluster)
  n143 = node-c288(w211) -> (w193:errorcluster)
  n144 = node-c288(w130) -> (w1:errorcluster)
  n145 = node-c288(w132) -> (w92:errorcluster)
  n146 = call-poly <vilib>:"CANopen Close.vi"("error in (no error)"=w143, "TPDO object in"=w158) -> ("error out"=w153:errorcluster)  [unwired: 9 in]
  n147 = call-poly <vilib>:"CANopen Close.vi"("error in (no error)"=w168, "TPDO object in"=w183) -> ("error out"=w178:errorcluster)  [unwired: 9 in]
  n148 = call-poly <vilib>:"CANopen Close.vi"("error in (no error)"=w193, "TPDO object in"=w208) -> ("error out"=w203:errorcluster)  [unwired: 9 in]
  n149 = call <vilib>:"CANopen NMT Write.vi"("node-ID (0)"="node-ID 3", "error in (no error)"=w153, "command"=w152, "interface object in"=w140) -> ("error out"=w155:errorcluster, "interface object out"=w154:refnum<k20>)  [unwired: 6 in]
  n150 = call <vilib>:"CANopen NMT Write.vi"("node-ID (0)"="node-ID 2", "error in (no error)"=w178, "command"=w177, "interface object in"=w165) -> ("error out"=w180:errorcluster, "interface object out"=w179:refnum<k20>)  [unwired: 6 in]
  n151 = call <vilib>:"CANopen NMT Write.vi"("node-ID (0)"="node-ID", "error in (no error)"=w203, "command"=w202, "interface object in"=w190) -> ("error out"=w205:errorcluster, "interface object out"=w204:refnum<k20>)  [unwired: 6 in]
  n152 = call-poly <vilib>:"CANopen Close.vi"("error in (no error)"=w155, "interface object in"=w154) -> ("error out"=w142:errorcluster)  [unwired: 9 in]
  n153 = call-poly <vilib>:"CANopen Close.vi"("error in (no error)"=w180, "interface object in"=w179) -> ("error out"=w167:errorcluster)  [unwired: 9 in]
  n154 = call-poly <vilib>:"CANopen Close.vi"("error in (no error)"=w205, "interface object in"=w204) -> ("error out"=w192:errorcluster)  [unwired: 9 in]
  n155 = call <vilib>:"Simple Error Handler.vi"("error in (no error)"=w142) -> ()  [unwired: 4 in, 5 out]
  n156 = call <vilib>:"Simple Error Handler.vi"("error in (no error)"=w167) -> ()  [unwired: 4 in, 5 out]
  n157 = call <vilib>:"Simple Error Handler.vi"("error in (no error)"=w192) -> ()  [unwired: 4 in, 5 out]
  n158 = call-poly <vilib>:"CANopen Close.vi"("error in (no error)"=w92, "SYNC object in"=w94) -> ("error out"=w71:errorcluster)  [unwired: 9 in]
  n159 = call-poly <vilib>:"CANopen Create.vi"("node-ID"="node-ID  2", "error in (no error)"=w1, "interface object in"=w17) -> ("error out"=w14:errorcluster, "SDO object out"=w16:refnum<k20>)  [unwired: 6 in, 1 out]
  n160 = call-poly <vilib>:"CANopen Create.vi"("node-ID"="node-ID  4", "error in (no error)"=w71, "interface object in"=w74) -> ("error out"=w70:errorcluster, "SDO object out"=w73:refnum<k20>)  [unwired: 6 in, 1 out]
  n161 = call-poly <vilib>:"CANopen SDO Write.vi"("I16 data"=i16 0, "error in (no error)"=w14, "object sub-index (0)"=u8 0 ("sub-index"), "object index"=u16 24642, "SDO object in"=w16) -> ("error out"=w13:errorcluster, "completion code"=→"completion code 5":u32, "SDO object out"=w15:refnum<k20>)  [unwired: 4 in]
  n162 = call-poly <vilib>:"CANopen SDO Write.vi"("I16 data"=i16 0, "error in (no error)"=w70, "object sub-index (0)"=u8 0 ("sub-index"), "object index"=u16 24642, "SDO object in"=w73) -> ("error out"=w69:errorcluster, "completion code"=→"completion code":u32, "SDO object out"=w72:refnum<k20>)  [unwired: 4 in]
  n163 = call-poly <vilib>:"CANopen Close.vi"("error in (no error)"=w13, "SDO object in"=w15) -> ("error out"=w12:errorcluster)  [unwired: 9 in]
  n164 = call-poly <vilib>:"CANopen Close.vi"("error in (no error)"=w69, "SDO object in"=w72) -> ("error out"=w68:errorcluster)  [unwired: 9 in]
  n165 = call-poly <vilib>:"CANopen Close.vi"("error in (no error)"=w12, "RPDO object in"=w18) -> ("error out"=w36:errorcluster)  [unwired: 9 in]
  n166 = call-poly <vilib>:"CANopen Close.vi"("error in (no error)"=w68, "RPDO object in"=w75) -> ("error out"=w96:errorcluster)  [unwired: 9 in]
  n167 = call-poly <vilib>:"CANopen Close.vi"("error in (no error)"=w36, "TPDO object in"=w37) -> ("error out"=w35:errorcluster)  [unwired: 9 in]
  n168 = call-poly <vilib>:"CANopen Close.vi"("error in (no error)"=w96, "TPDO object in"=w97) -> ("error out"=w95:errorcluster)  [unwired: 9 in]
  n169 = call <vilib>:"CANopen NMT Write.vi"("node-ID (0)"="node-ID  2", "error in (no error)"=w35, "command"=w38, "interface object in"=w17) -> ("error out"=w40:errorcluster, "interface object out"=w39:refnum<k20>)  [unwired: 6 in]
  n170 = call <vilib>:"CANopen NMT Write.vi"("node-ID (0)"="node-ID  4", "error in (no error)"=w95, "command"=w98, "interface object in"=w74) -> ("error out"=w100:errorcluster, "interface object out"=w99:refnum<k20>)  [unwired: 6 in]
  n171 = call-poly <vilib>:"CANopen Close.vi"("error in (no error)"=w40, "interface object in"=w39) -> ("error out"=w34:errorcluster)  [unwired: 9 in]
  n172 = call-poly <vilib>:"CANopen Close.vi"("error in (no error)"=w100, "interface object in"=w99) -> ("error out"=w93:errorcluster)  [unwired: 9 in]
  n173 = call <vilib>:"Simple Error Handler.vi"("error in (no error)"=w34) -> ()  [unwired: 4 in, 5 out]
  n174 = call <vilib>:"Simple Error Handler.vi"("error in (no error)"=w93) -> ()  [unwired: 4 in, 5 out]
